vi "HCCDiceTester.vi"(11 "COM Port MicroZed":refnum<visa-resource-name>="COM4") -> ()   [LabVIEW 2014]
uses:
  c_StateMachine_States.ctl
  <vilib>/vision/Vision Builder AI/API.llb/IVB Interface - VBAI Version.ctl
  c_VBAI_SelcectInspection.ctl
  c_PlatePosEnum.ctl
  c_InstructionEnum.ctl
  c_Calib_States.ctl
  c_ShowCorner_States.ctl
  c_FindReference_States.ctl
  c_ReportMessages.ctl
  g_Stop.vi
  g_ReportControl.vi
  g_GPCounters.vi
  g_CipHolderConstants.vi
  g_CommandParam.vi
  g_VBAIMeasurements.vi
  g_MicroZed_Interface.vi
  g_ChipData.vi
  g_ImageCalibration.vi
  g_HCCConstants.vi
panel:
  in  "RedoAlignment":bool
  out "Chip Y":dbl
  out "Chip X":dbl
  in  "BrightnessAdjustment":bool
  in  "Move Plate":bool
  out "Alignment Successful":bool
  in  "CancelAlignment":bool
  in  "ConfirmAlignment":bool
  in  "ProbecardOK":bool
  out "ChipsComplete":bool
  out "LoopBreak":bool
  in  "ImageBusy":bool
  in  "stop":bool
  out "Image":T1(plugin-control)
  out "Actual State":T2
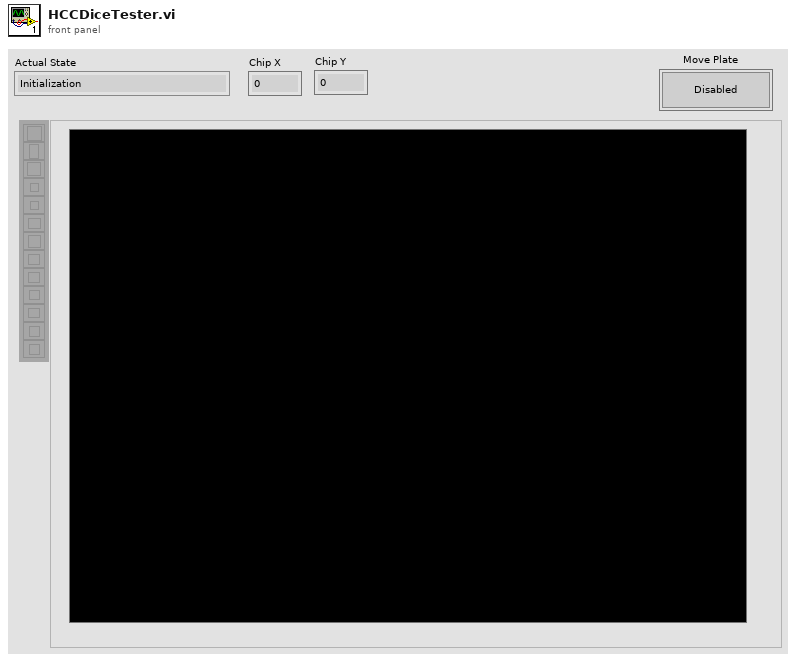
[diagram p1: front panel]
types:
  T1 = typedef "IMAQ Image.ctl" = refnum<image>
  T2 = typedef "c_StateMachine_States.ctl" = enum16{"Initialization", "Load", "Calibration", "Next Slot", "Chip Alignment", "Test", "Report", "End"}
  T3 = enum8{"Enabled", "Disabled", "Disabled and Grayed Out"}
  T4 = typedef "IVB Interface - VBAI Version.ctl" = u16
  T5 = enum32{"invalid app kind", "Development System", "Run Time System", "Student Edition", "Embedded LabVIEW", "Evaluation", "Custom"}
  T6 = typedef "VBAIInterface.ctl" = refnum<k21>
  T7 = typedef "c_InstructionEnum.ctl" = enum16{"Move Absolute", "Increment", "Move Home", "Motion Kill", "Move Plate", "Set Stepsize", "Query Position"}
  T8 = typedef "c_PlatePosEnum.ctl" = enum16{"Contact", "Seperate"}
  T9 = typedef "c_VBAI_SelcectInspection.ctl" = enum16{"Image Acquisition", "Find Reference", "Chip Alignment", "Adjustment", "Porbecard Positioning"}
  T10 = typedef "c_Calib_States.ctl" = enum16{"Find Top", "Show Corners", "Find Reference"}
  T11 = typedef "c_ShowCorner_States.ctl" = enum16{"Intruction", "Set Increment", "First Move Right", "Move Right", "Move Left", "Confirm"}
  T12 = typedef "c_FindReference_States.ctl" = enum16{"Move to Side", "Settings", "Find Chipslot", "Make Step", "Set Reference"}
  T13 = typedef "c_ReportMessages.ctl" = string
  T14 = cluster{"PASS/FAIL Flag":bool, "Numeric Measurement":dbl, "String Measurement":string, "Report Text":string}
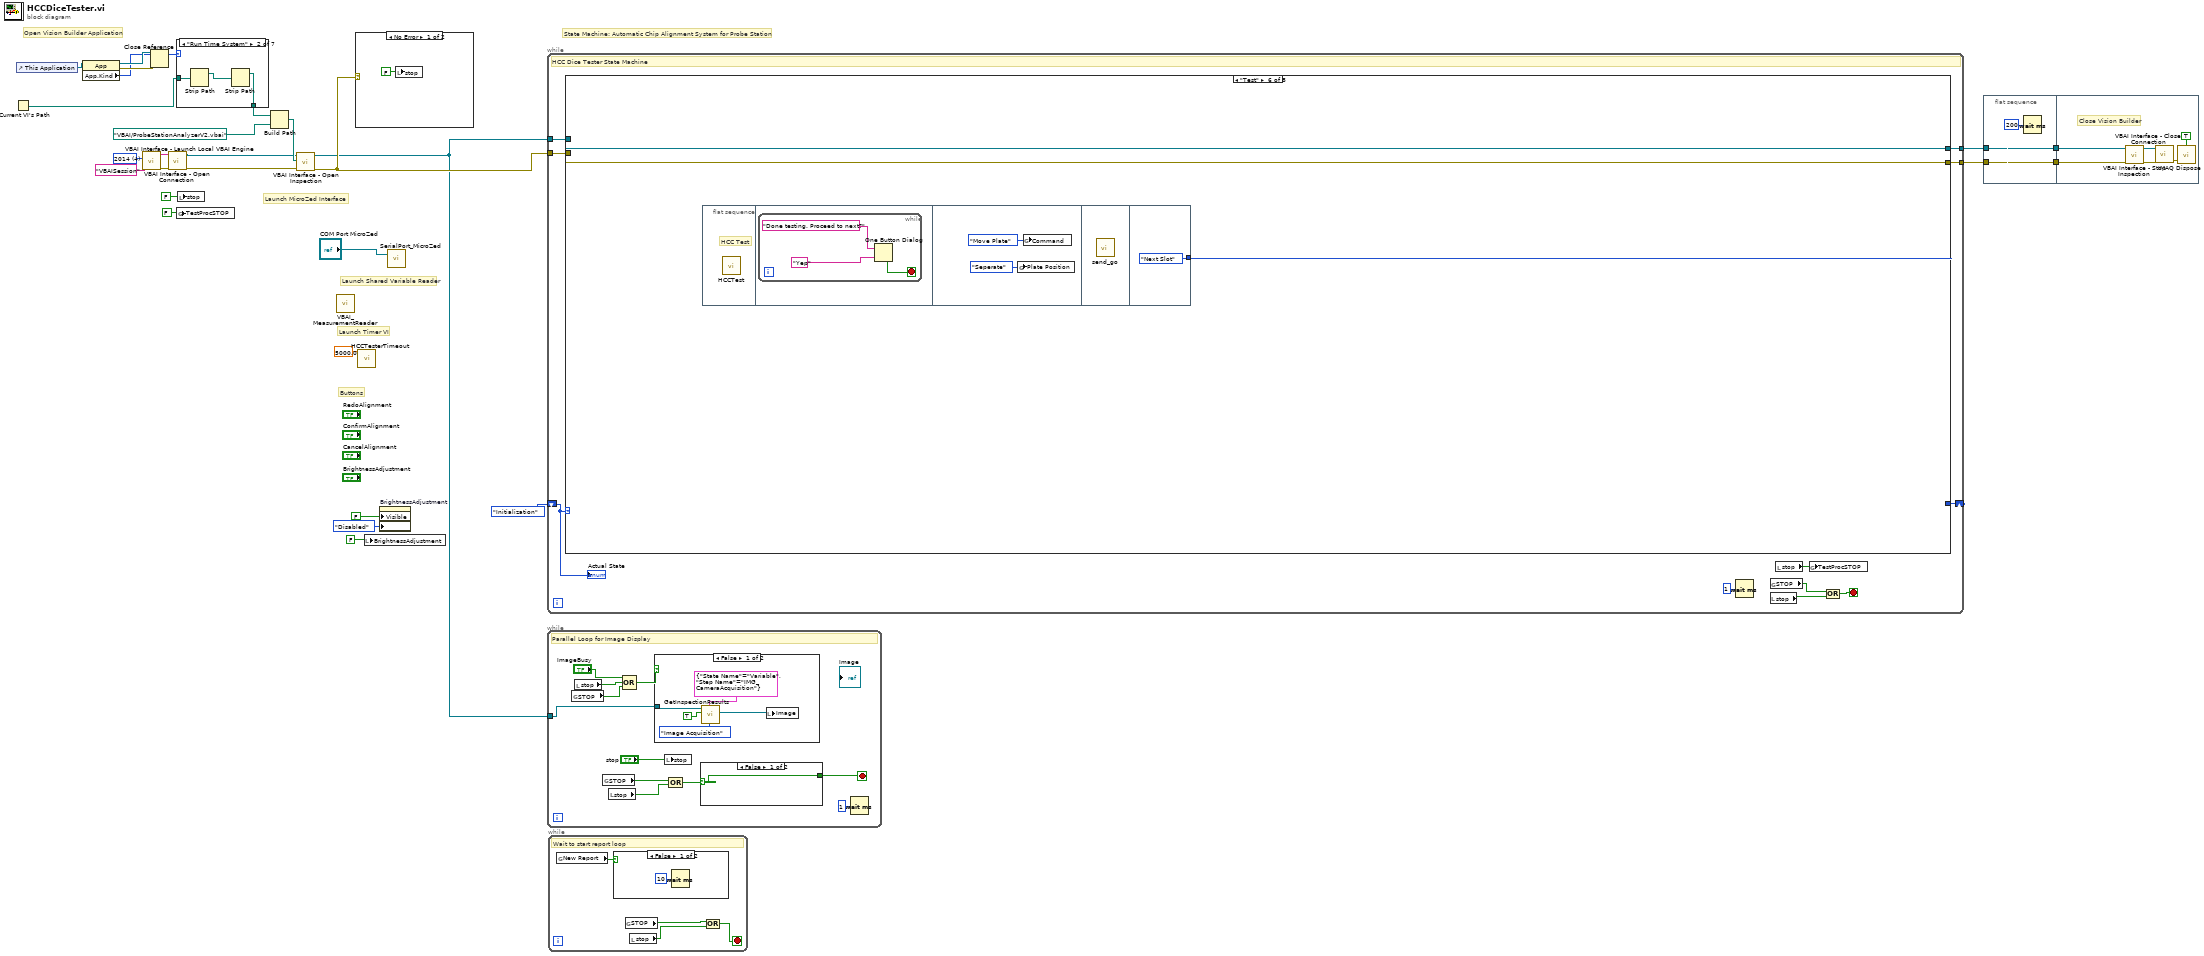
[diagram p0: block diagram]
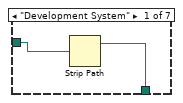
[diagram p2: hidden frame]
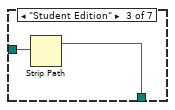
[diagram p3: hidden frame]
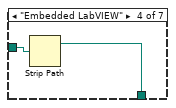
[diagram p4: hidden frame]
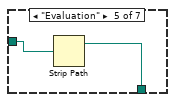
[diagram p5: hidden frame]
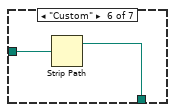
[diagram p6: hidden frame]
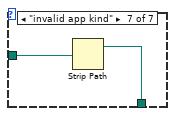
[diagram p7: hidden frame]
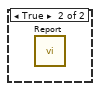
[diagram p8: hidden frame]
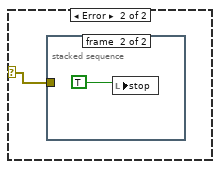
[diagram p9: hidden frame]
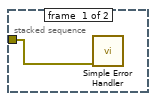
[diagram p10: hidden frame]
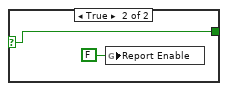
[diagram p11: hidden frame]
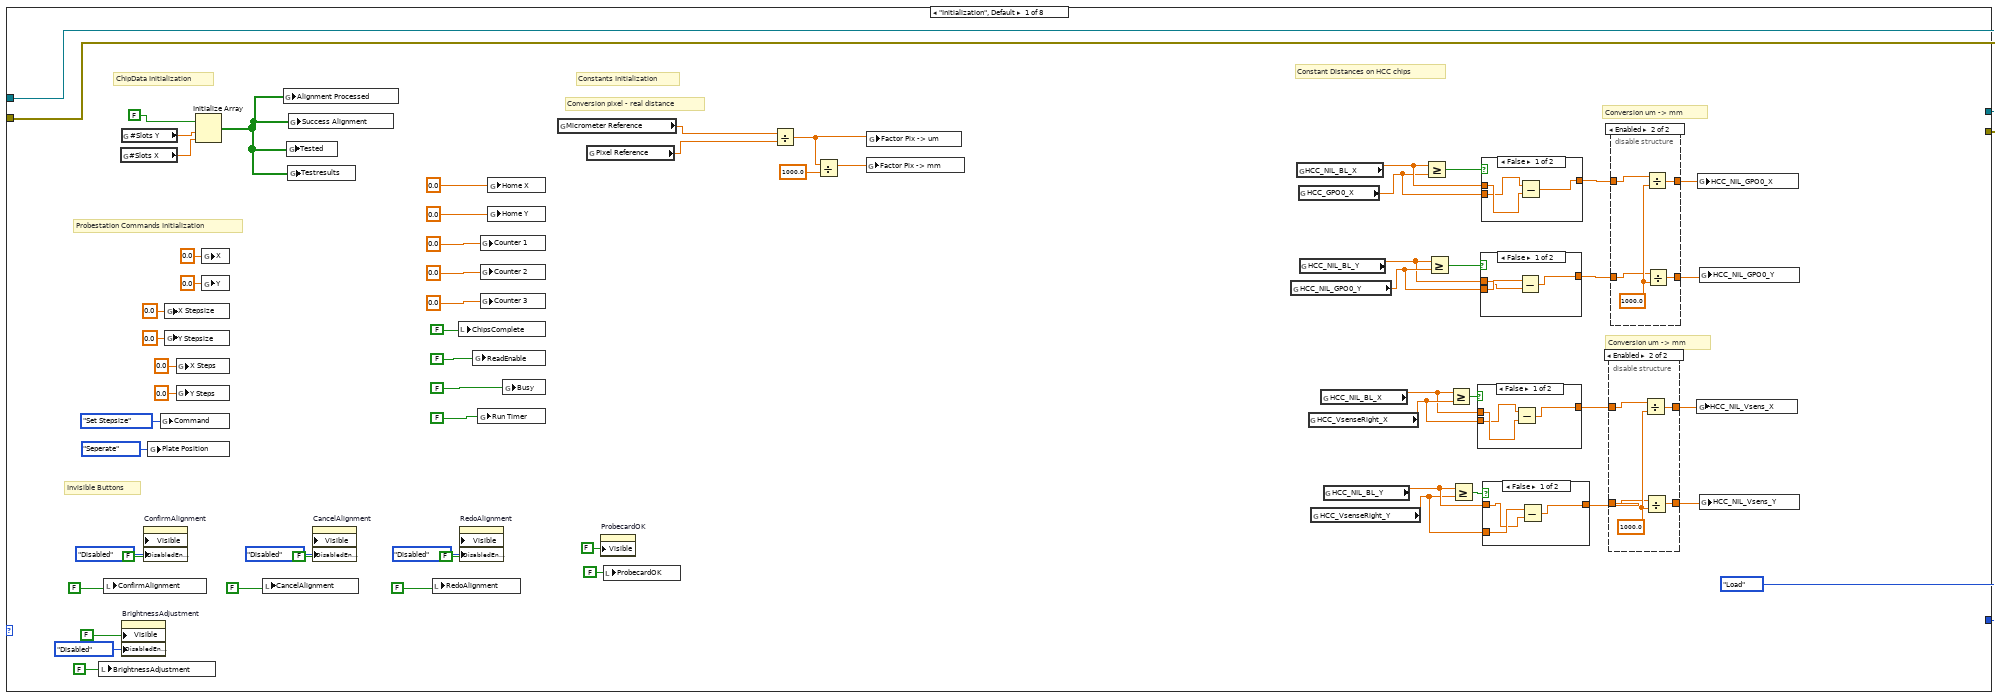
[diagram p13: hidden frame]
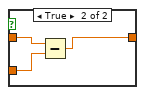
[diagram p15: hidden frame]
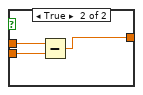
[diagram p16: hidden frame]
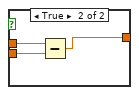
[diagram p18: hidden frame]
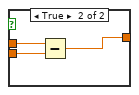
[diagram p19: hidden frame]
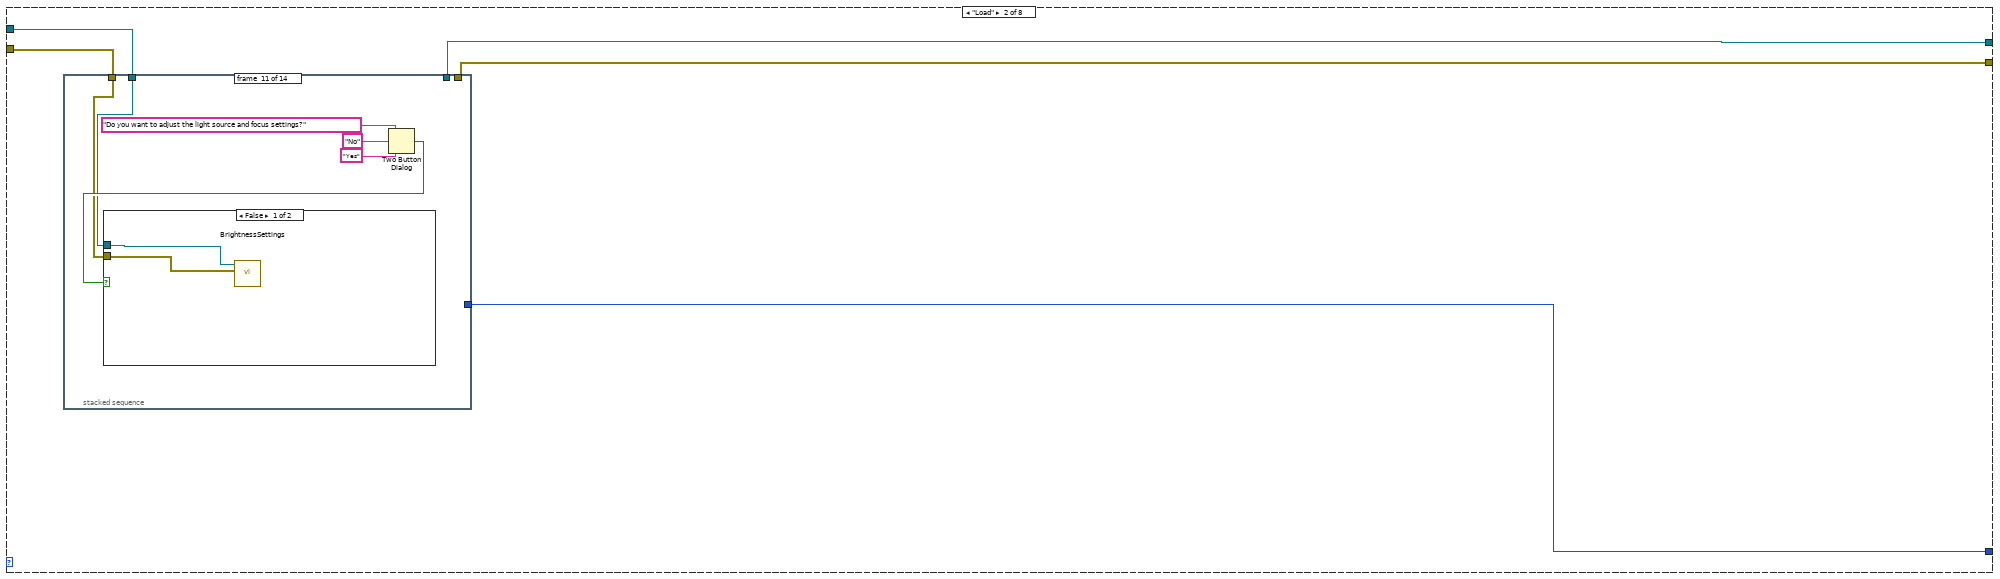
[diagram p20: hidden frame]
diagram:
  w27 = T4 4 items=["2010", "2011", "2012", "2013", "2014"] ("Engine Version")
  # "Buttons"
  # "Launch Timer VI"
  # "Launch Shared Variable Reader"
  # "Launch MicroZed Interface"
  # "Open Vision Builder Application"
  # "State Machine: Automatic Chip Alignment System for Probe Station"
  n1 = Current VI's Path() -> (path=w5:path)
  n2 = control-ref of="This Application"() -> (w7:refnum<vi>)
  n3 = property class="App"(reference=w7) -> (reference out=w9:refnum<vi>, error out=w8:errorcluster, "App.Kind"=w6:T5)  [unwired: 1 in]
  n4 = call <vilib>:"VBAI Interface - Launch Local VBAI Engine.vi"("Engine Version"=w27, "Local VBAI Engine Name"="VBAISession") -> ("error out"=w26:errorcluster, "Session Name Out"=w25:string)  [unwired: 8 in]
  n5 = Close Reference(reference=w9, error in (no error)=w8) -> ()  [unwired: 1 out]
  n6 = call <vilib>:"VBAI Interface - Open Connection.vi"("error in"=w26, "Session In"=w25) -> ("error out"=w20:errorcluster, "Session Out"=w21:T6)  [unwired: 8 in]
  n7 = case shown="\"Run Time System\"" w6 {
    tunnel: w5 -> [w30 w33 w35 w37 w39 w41 w42]
    tunnel: [w29 w31 w34 w36 w38 w40 w43] -> w4
    frame "Development System" {
      n8 = Strip Path(path=w30) -> (stripped path=w29:path)  [unwired: 1 out]
    }
    frame "Run Time System" {
      n9 = Strip Path(path=w33) -> (stripped path=w32:path)  [unwired: 1 out]
      n10 = Strip Path(path=w32) -> (stripped path=w31:path)  [unwired: 1 out]
    }
    frame "Student Edition" {
      n11 = Strip Path(path=w35) -> (stripped path=w34:path)  [unwired: 1 out]
    }
    frame "Embedded LabVIEW" {
      n12 = Strip Path(path=w37) -> (stripped path=w36:path)  [unwired: 1 out]
    }
    frame "Evaluation" {
      n13 = Strip Path(path=w39) -> (stripped path=w38:path)  [unwired: 1 out]
    }
    frame "Custom" {
      n14 = Strip Path(path=w41) -> (stripped path=w40:path)  [unwired: 1 out]
    }
    frame "invalid app kind" {
      n15 = Strip Path(path=w42) -> (stripped path=w43:path)  [unwired: 1 out]
    }
  }
  n16 = global write "g_Stop.vi" "TestProcSTOP"(FALSE ("TestProcSTOP")) -> ()
  n17 = local write "stop"(FALSE ("stop")) -> ()
  n18 = Build Path(base path=w4, name or relative path=path "VBAI/ProbeStationAnalyzerV2.vbai") -> (appended path=w22:path)
  n19 = call <vilib>:"VBAI Interface - Open Inspection.vi"("error in"=w20, "Path"=w22, "Session In"=w21) -> ("error out"=w17:errorcluster, "Session Out"=w16:T6)  [unwired: 7 in]
  n20 = call "VBAI_MeasurementReader.vi"() -> ()  [unwired: 12 in]
  n21 = case shown="No Error" w17 {
    selector: w17 -> [_ w45]
    frame No Error {
      n22 = local write "stop"(FALSE) -> ()
    }
    frame Error {
      n23 = stacked-sequence {
        tunnel: w45 -> [w46 _]
        frame #0 {
          n24 = call <vilib>:"Simple Error Handler.vi"("error in (no error)"=w46) -> ()  [unwired: 4 in, 5 out]
        }
        frame #1 {
          n25 = local write "stop"(TRUE) -> ()
        }
      }
    }
  }
  n26 = call "HCCTesterTimeout.vi"("Timeout"=5000.0) -> ()  [unwired: 11 in]
  n27 = local write "BrightnessAdjustment"(FALSE ("CancelAlignment")) -> ()
  n28 = property on="BrightnessAdjustment" class="Bool (strict)"("Visible"=FALSE, "DisabledEnum"=T3."Disabled" ("Disabled")) -> ()  [unwired: 2 in, 2 out]
  n29 = call "SerialPort_MicroZed.vi"("COM Port"="COM Port MicroZed") -> ()  [unwired: 2 in, 1 out]
  n30 = while {
    shift-right: [w58] -> _
    shift-left: c_StateMachine_States."Initialization" -> [w48]
    tunnel: w16 -> [w54]
    tunnel: w17 -> [w52]
    tunnel: [w55] -> w19
    tunnel: [w53] -> w18
    stop <- w56 stop-if-true
    # "HCC Dice Tester State Machine"
    n31 = case shown="\"Test\"" w48 {
      tunnel: [c_StateMachine_States."Load" w164 c_StateMachine_States."Next Slot" w433 w499 w639 c_StateMachine_States."End" c_StateMachine_States."End"] -> w58
      tunnel: [w67 w161 w207 w435 w503 w641 w651 w664] -> w55
      tunnel: w54 -> [w67 w162 w209 w435 w505 w641 w651 w664]
      tunnel: [w66 w160 w206 w434 w502 w640 w650 w663] -> w53
      tunnel: w52 -> [w66 w163 w208 w434 w504 w640 w650 w663]
      frame "Initialization", Default {
        # "Constant Distances on HCC chips"
        # "Invisible Buttons"
        # "Conversion pixel - real distance"
        # "Probestation Commands Initialization"
        # "Conversion um -> mm"
        # "Conversion um -> mm"
        # "Constants Initialization"
        # "ChipData Initialization"
        n32 = local write "BrightnessAdjustment"(FALSE ("CancelAlignment")) -> ()
        n33 = local write "ConfirmAlignment"(FALSE ("ConfirmAlignment")) -> ()
        n34 = global read "g_CipHolderConstants.vi" "#Slots X"() -> (w120:dbl)
        n35 = global read "g_CipHolderConstants.vi" "#Slots Y"() -> (w121:dbl)
        n36 = property on="BrightnessAdjustment" class="Bool (strict)"("Visible"=FALSE, "DisabledEnum"=T3."Disabled" ("Disabled")) -> ()  [unwired: 2 in, 2 out]
        n37 = property on="ConfirmAlignment" class="Bool (strict)"("Visible"=FALSE, "DisabledEnum"=T3."Disabled" ("Disabled")) -> ()  [unwired: 2 in, 2 out]
        n38 = global write "g_CommandParam.vi" "Plate Position"(c_PlatePosEnum."Seperate" ("Plate Position")) -> ()
        n39 = global write "g_CommandParam.vi" "Command"(c_InstructionEnum."Set Stepsize" ("Command")) -> ()
        n40 = global write "g_CommandParam.vi" "X Stepsize"(0.0 ("X Stepsize")) -> ()
        n41 = global write "g_CommandParam.vi" "Y Stepsize"(0.0 ("Y Stepsize")) -> ()
        n42 = global write "g_CommandParam.vi" "X Steps"(0.0 ("X Steps")) -> ()
        n43 = global write "g_CommandParam.vi" "Y Steps"(0.0 ("Y Steps")) -> ()
        n44 = Initialize Array(FALSE, w121, w120) -> (w79:bool[][])
        n45 = global write "g_CommandParam.vi" "X"(0.0 ("X")) -> ()
        n46 = global write "g_CommandParam.vi" "Y"(0.0 ("Y")) -> ()
        n47 = local write "CancelAlignment"(FALSE ("CancelAlignment")) -> ()
        n48 = global write "g_ChipData.vi" "Alignment Processed"(w79) -> ()
        n49 = global write "g_ChipData.vi" "Tested"(w79) -> ()
        n50 = global write "g_ChipData.vi" "Testresults"(w79) -> ()
        n51 = global write "g_ChipData.vi" "Success Alignment"(w79) -> ()
        n52 = property on="CancelAlignment" class="Bool (strict)"("Visible"=FALSE, "DisabledEnum"=T3."Disabled" ("Disabled")) -> ()  [unwired: 2 in, 2 out]
        n53 = local write "RedoAlignment"(FALSE ("CancelAlignment")) -> ()
        n54 = local write "ChipsComplete"(FALSE ("ChipsComplete")) -> ()
        n55 = property on="RedoAlignment" class="Bool (strict)"("Visible"=FALSE ("RedoAlignment"), "DisabledEnum"=T3."Disabled" ("RedoAlignment")) -> ()  [unwired: 2 in, 2 out]
        n56 = global write "g_VBAIMeasurements.vi" "ReadEnable"(FALSE ("SharedVariableReadEnable")) -> ()
        n57 = global write "g_MicroZed_Interface.vi" "Run Timer"(FALSE ("Start")) -> ()
        n58 = global write "g_GPCounters.vi" "Counter 1"(0.0 ("Counter 1")) -> ()
        n59 = global write "g_GPCounters.vi" "Counter 2"(0.0 ("Counter 1")) -> ()
        n60 = global write "g_GPCounters.vi" "Counter 3"(0.0 ("Counter 1")) -> ()
        n61 = global write "g_CipHolderConstants.vi" "Home X"(0.0 ("Home X")) -> ()
        n62 = global write "g_CipHolderConstants.vi" "Home Y"(0.0 ("Home X")) -> ()
        n63 = global write "g_MicroZed_Interface.vi" "Busy"(FALSE ("Busy")) -> ()
        n64 = global read "g_ImageCalibration.vi" "Micrometer Reference"() -> (w111:dbl)
        n65 = global read "g_ImageCalibration.vi" "Pixel Reference"() -> (w112:dbl)
        n66 = property on="ProbecardOK" class="Bool (strict)"("Visible"=FALSE) -> ()  [unwired: 2 in, 2 out]
        n67 = local write "ProbecardOK"(FALSE ("ProbecardOK")) -> ()
        n68 = Divide(x=w111, y=w112) -> (x/y=w110:dbl)
        n69 = Divide(x=w110, y=1000.0) -> (x/y=w108:dbl)
        n70 = global write "g_ImageCalibration.vi" "Factor Pix -> mm"(w108) -> ()
        n71 = global write "g_ImageCalibration.vi" "Factor Pix -> um"(w110) -> ()
        n72 = global read "g_HCCConstants.vi" "HCC_NIL_GPO0_Y"() -> (w104:dbl)
        n73 = global read "g_HCCConstants.vi" "HCC_NIL_BL_X"() -> (w106:dbl)
        n74 = global read "g_HCCConstants.vi" "HCC_GPO0_X"() -> (w105:dbl)
        n75 = global read "g_HCCConstants.vi" "HCC_NIL_BL_Y"() -> (w103:dbl)
        n76 = global read "g_HCCConstants.vi" "HCC_VsenseRight_X"() -> (w90:dbl)
        n77 = global read "g_HCCConstants.vi" "HCC_VsenseRight_Y"() -> (w91:dbl)
        n78 = global read "g_HCCConstants.vi" "HCC_NIL_BL_X"() -> (w89:dbl)
        n79 = global read "g_HCCConstants.vi" "HCC_NIL_BL_Y"() -> (w92:dbl)
        n80 = Greater Or Equal?(x=w106, y=w105) -> (x >= y?=w107:bool)
        n81 = Greater Or Equal?(x=w103, y=w104) -> (x >= y?=w102:bool)
        n82 = Greater Or Equal?(x=w89, y=w90) -> (x >= y?=w88:bool)
        n83 = Greater Or Equal?(x=w92, y=w91) -> (x >= y?=w93:bool)
        n84 = case shown="False" w88 {
          tunnel: w89 -> [w136 w140]
          tunnel: w90 -> [w135 w139]
          tunnel: [w137 w138] -> w94
          frame False {
            n85 = Subtract(x=w135, y=w136) -> (x-y=w137:dbl)
          }
          frame True {
            n86 = Subtract(x=w140, y=w139) -> (x-y=w138:dbl)
          }
        }
        n87 = case shown="False" w102 {
          tunnel: w103 -> [w148 w153]
          tunnel: w104 -> [w149 w152]
          tunnel: [w150 w151] -> w99
          frame False {
            n88 = Subtract(x=w149, y=w148) -> (x-y=w150:dbl)
          }
          frame True {
            n89 = Subtract(x=w153, y=w152) -> (x-y=w151:dbl)
          }
        }
        n90 = case shown="False" w107 {
          tunnel: w106 -> [w155 w159]
          tunnel: w105 -> [w154 w158]
          tunnel: [w156 w157] -> w101
          frame False {
            n91 = Subtract(x=w154, y=w155) -> (x-y=w156:dbl)
          }
          frame True {
            n92 = Subtract(x=w159, y=w158) -> (x-y=w157:dbl)
          }
        }
        n93 = case shown="False" w93 {
          tunnel: w92 -> [w129 w133]
          tunnel: w91 -> [w130 w132]
          tunnel: [w131 w134] -> w96
          frame False {
            n94 = Subtract(x=w130, y=w129) -> (x-y=w131:dbl)
          }
          frame True {
            n95 = Subtract(x=w133, y=w132) -> (x-y=w134:dbl)
          }
        }
        n96 = disable-structure shown="Enabled" {
          disable-tunnel: w94 -> [w123 w125]
          disable-tunnel: [w123 w128] -> w95
          disable-tunnel: w96 -> [w122 w124]
          disable-tunnel: [w122 w127] -> w97
          frame Disabled {
          }
          frame Enabled {
            w126 = 1000.0 ("y")
            n97 = Divide(x=w125, y=w126) -> (x/y=w128:dbl)
            n98 = Divide(x=w124, y=w126) -> (x/y=w127:dbl)
          }
        }
        n99 = disable-structure shown="Enabled" {
          disable-tunnel: w101 -> [w142 w144]
          disable-tunnel: [w142 w147] -> w100
          disable-tunnel: w99 -> [w141 w143]
          disable-tunnel: [w141 w146] -> w98
          frame Disabled {
          }
          frame Enabled {
            w145 = 1000.0 ("y")
            n100 = Divide(x=w144, y=w145) -> (x/y=w147:dbl)
            n101 = Divide(x=w143, y=w145) -> (x/y=w146:dbl)
          }
        }
        n102 = global write "g_HCCConstants.vi" "HCC_NIL_Vsens_X"(w95) -> ()
        n103 = global write "g_HCCConstants.vi" "HCC_NIL_GPO0_X"(w100) -> ()
        n104 = global write "g_HCCConstants.vi" "HCC_NIL_GPO0_Y"(w98) -> ()
        n105 = global write "g_HCCConstants.vi" "HCC_NIL_Vsens_Y"(w97) -> ()
      }
      frame "Load" {
        n106 = stacked-sequence {
          tunnel: w162 -> [_ _ _ _ _ _ _ _ w179 _ w194 _ _ _]
          tunnel: w163 -> [_ _ _ _ _ _ _ _ w178 _ w193 _ _ _]
          tunnel: [_ _ _ _ _ _ _ _ _ _ _ _ _ c_StateMachine_States."Calibration"] -> w164
          tunnel: [_ _ _ _ _ _ _ _ w177 _ _ _ _ _] -> w161
          tunnel: [_ _ _ _ _ _ _ _ w176 _ _ _ _ _] -> w160
          frame #0 {
            n107 = global write "g_CommandParam.vi" "Command"(c_InstructionEnum."Move Absolute" ("Command")) -> ()
            n108 = call "send_go.vi"() -> ()  [unwired: 12 in]
            n109 = global write "g_CommandParam.vi" "X"(0.0 ("X")) -> ()
            n110 = global write "g_CommandParam.vi" "Y"(70.0 ("Y")) -> ()
          }
          frame #1 {
            n111 = One Button Dialog(message="Place the Chips on the Chipholder and click OK") -> ()  [unwired: 1 in, 1 out]
          }
          frame #2 {
            # "Select the chipslots that are\noccupied by a chip"
            n112 = call "ChipSlotSelect.vi"() -> ()  [unwired: 12 in]
          }
          frame #3 {
            # "Start a new report dialog"
            n113 = global write "g_ReportControl.vi" "New Report"(TRUE ("New Report")) -> ()
          }
          frame #4 {
            n114 = Wait (ms)(milliseconds to wait=u32 1) -> ()  [unwired: 1 out]
          }
          frame #5 {
            # "Wait until new report dialog ended"
            n115 = while {
              stop <- w172 stop-if-true
              n116 = global read "g_ReportControl.vi" "New Report"() -> (w173:bool)
              n117 = Not(x=w173) -> (.not. x?=w172:bool)
              n118 = Wait (ms)(milliseconds to wait=u32 100) -> ()  [unwired: 1 out]
            }
          }
          frame #6 {
            # "Set the Configurationregisters\nfor the HCC chips"
            n119 = call "HCCConfig.vi"() -> ()  [unwired: 12 in]
          }
          frame #7 {
            # "Propare for Image Processing\n- Set Image Busy\n- Make Button visible for\nProbecard Alignment Confirm"
            n120 = local write "ImageBusy"(TRUE ("ImageBusy")) -> ()
            n121 = property on="ProbecardOK" class="Bool (strict)"("Visible"=TRUE) -> ()  [unwired: 2 in, 2 out]
          }
          frame #8 {
            # "Show Probecard Highlight until Confirm"
            n122 = while {
              tunnel: [w189] -> w177
              tunnel: w178 -> [w182]
              tunnel: [w188] -> w176
              tunnel: w179 -> [w183]
              stop <- w185 stop-if-true
              n123 = global read "g_Stop.vi" "TestProcSTOP"() -> (w187:bool)
              n124 = global read "g_Stop.vi" "STOP"() -> (w186:bool)
              n125 = call "GetInspectionResults.vi"("Select Inspection"=c_VBAI_SelcectInspection."Porbecard Positioning" ("Enum"), "Image Step Name (default last image used by inspection)"=cluster{"State Name":string, "Step Name":string} {"State Name"="Variable", "Step Name"="IMG_ProbeCardPosition"}, "error in (no error)"=w182, "Image Enable"=TRUE, "Refnum in"=w183) -> ("error out"=w188:errorcluster, "Image Dst Out"=w181:T1, "Refnum out"=w189:T6)  [unwired: 2 in, 2 out]
              n126 = Compound Arithmetic op=OR("ProbecardOK", w186, w187) -> (w185:bool)
              n127 = local write "Image"(w181) -> ()
            }
          }
          frame #9 {
            # "Hide Button again and\nfree image for normal Display"
            n128 = property on="ProbecardOK" class="Bool (strict)"("Visible"=FALSE) -> ()  [unwired: 2 in, 2 out]
          }
          frame #10 {
            n129 = Two Button Dialog(message="Do you want to adjust the light source and focus settings?", 1:"Yes" ("F button name (\"Cancel\")"), 2:"No" ("T button name (\"OK\")")) -> (T button?=w195:bool)
            n130 = case shown="False" w195 {
              tunnel: w194 -> [w200 _]
              tunnel: w193 -> [w199 _]
              frame False {
                n131 = call "BrightnessSettings.vi"("error in (no error)"=w199, "Refnum in"=w200) -> ()  [unwired: 8 in, 2 out]
              }
              frame True {
              }
            }
          }
          frame #11 {
            n132 = Wait (ms)(milliseconds to wait=u32 100) -> ()  [unwired: 1 out]
          }
          frame #12 {
            n133 = disable-structure shown="Disabled" {
              frame Disabled {
                n134 = local write "ImageBusy"(FALSE ("ImageBusy")) -> ()
              }
              frame Enabled {
              }
            }
          }
          frame #13 {
          }
        }
      }
      frame "Calibration" {
        n135 = while {
          shift-right: [w210] -> _
          shift-left: c_Calib_States."Find Top" -> [w213]
          tunnel: w209 -> [w218]
          tunnel: w208 -> [w217]
          tunnel: [w216] -> w207
          tunnel: [w215] -> w206
          stop <- w214 stop-if-true
          # "Calibration State Machine"
          n136 = case shown="\"Find Reference\"" w213 {
            tunnel: [FALSE FALSE TRUE] -> w211
            tunnel: [w223 c_Calib_States."Find Reference" c_Calib_States."Find Reference"] -> w210
            tunnel: w218 -> [w225 w288 w341]
            tunnel: w217 -> [w224 w290 w340]
            tunnel: [w222 w288 w338] -> w216
            tunnel: [w221 w290 w337] -> w215
            frame "Find Top", Default {
              n137 = stacked-sequence {
                tunnel: w225 -> [_ _ _ _ _ _ w248 _]
                tunnel: w224 -> [_ _ _ _ _ _ w247 _]
                tunnel: [_ _ _ _ _ _ w246 _] -> w222
                tunnel: [_ _ _ _ _ _ w245 _] -> w221
                tunnel: [_ _ _ _ _ _ _ c_Calib_States."Show Corners"] -> w223
                frame #0 {
                  n138 = Wait (ms)(milliseconds to wait=u32 1) -> ()  [unwired: 1 out]
                }
                frame #1 {
                  # "Move back from the Load Position towards the\nregion of the chipholder"
                  n139 = global read "g_CipHolderConstants.vi" "Length Chipslot"() -> (w232:dbl)
                  n140 = global read "g_CipHolderConstants.vi" "#Slots Y"() -> (w231:dbl)
                  n141 = global write "g_CommandParam.vi" "Command"(c_InstructionEnum."Move Absolute" ("Command")) -> ()
                  n142 = global write "g_CommandParam.vi" "X"(0.0 ("X")) -> ()
                  n143 = Multiply(x=w231, y=w232) -> (x*y=w233:dbl)
                  n144 = Divide(x=w233, y=2.0) -> (x/y=w230:dbl)
                  n145 = Multiply(x=w230, y=1.0) -> (x*y=w229:dbl)
                  n146 = global write "g_CommandParam.vi" "Y"(w229) -> ()
                }
                frame #2 {
                  # "Send Command"
                  n147 = call "send_go.vi"() -> ()  [unwired: 12 in]
                }
                frame #3 {
                  # "Wait during movement"
                  n148 = Wait (ms)(milliseconds to wait=u32 1500) -> ()  [unwired: 1 out]
                }
                frame #4 {
                  # "Wait until Probestation is ready"
                  n149 = call "PS_Ready.vi"("WaitForReady"=TRUE) -> ()  [unwired: 10 in, 1 out]
                }
                frame #5 {
                  n150 = flat-sequence {
                    frame #0 {
                      # "Prepare to find Top Edge\n- Set Stepsize\n- Set Image Busz for Image Processing\n- Set maximal Stepcounter to 0"
                      n151 = global write "g_GPCounters.vi" "Counter 2"(0.0 ("Counter 2")) -> ()
                      n152 = global write "g_CommandParam.vi" "Y Stepsize"(0.1 ("Y Stepsize")) -> ()
                      n153 = local write "ImageBusy"(TRUE ("ImageBusy")) -> ()
                      n154 = global write "g_CommandParam.vi" "X Stepsize"(0.1 ("X Stepsize")) -> ()
                      n155 = global write "g_CommandParam.vi" "Command"(c_InstructionEnum."Set Stepsize" ("Command")) -> ()
                    }
                    frame #1 {
                    }
                    frame #2 {
                      n156 = call "send_go.vi"() -> ()  [unwired: 12 in]
                    }
                    frame #3 {
                      n157 = call "send_go.vi"() -> ()  [unwired: 12 in]
                    }
                    frame #4 {
                      n158 = Wait (ms)(milliseconds to wait=u32 1) -> ()  [unwired: 1 out]
                    }
                  }
                }
                frame #6 {
                  n159 = while {
                    tunnel: w248 -> [w264]
                    tunnel: w247 -> [w263]
                    tunnel: [w262] -> w246
                    tunnel: [w261] -> w245
                    stop <- w269 stop-if-true
                    # "Stops the Loop when more than 50 moves executed\nchange steps from 40 to 50 8/19/15 -nl"
                    # "Edge Detection\nLooking for Top Edge of \nthe Chipholder"
                    # "This Loop moves the chuck until the top edge of the chipholder is detected"
                    n160 = call "GetInspectionResults.vi"("Select Inspection"=c_VBAI_SelcectInspection."Find Reference", "Image Step Name (default last image used by inspection)"=cluster{"State Name":string, "Step Name":string} {"State Name"="Variable", "Step Name"="IMG_EdgeFinder"}, "error in (no error)"=w263, "StepName"="FindTop", "Image Enable"=TRUE, "Refnum in"=w264) -> ("error out"=w261:errorcluster, "Results"=w267:T14, "Image Dst Out"=w260:T1, "Refnum out"=w262:T6)  [unwired: 1 in, 1 out]
                    n161 = local write "Image"(w260) -> ()
                    n162 = Unbundle By Name(w267) -> ("PASS/FAIL Flag"=w250:bool)
                    n163 = case shown="False" w250 {
                      frame False {
                        # "If no Edge detected -> Move a step"
                        n164 = stacked-sequence {
                          frame #0 {
                            n165 = global read "g_GPCounters.vi" "Counter 2"() -> (w274:dbl)
                            n166 = global write "g_GPCounters.vi" "Counter 1"(0.0 ("Counter 1")) -> ()
                            n167 = Increment(x=w274) -> (x+1=w275:dbl)
                            n168 = global write "g_GPCounters.vi" "Counter 2"(w275) -> ()
                          }
                          frame #1 {
                            n169 = global write "g_CommandParam.vi" "Y Stepsize"(0.1 ("Y Stepsize")) -> ()
                            n170 = global write "g_CommandParam.vi" "X Stepsize"(0.1 ("X Stepsize")) -> ()
                            n171 = global write "g_CommandParam.vi" "Command"(c_InstructionEnum."Set Stepsize" ("Command")) -> ()
                          }
                          frame #2 {
                            n172 = call "send_go.vi"() -> ()  [unwired: 12 in]
                          }
                          frame #3 {
                            n173 = global write "g_CommandParam.vi" "Y Steps"(-1.0 ("Y Stepsize")) -> ()
                            n174 = global write "g_CommandParam.vi" "X Steps"(0.0 ("X Stepsize")) -> ()
                            n175 = global write "g_CommandParam.vi" "Command"(c_InstructionEnum."Increment" ("Command")) -> ()
                          }
                          frame #4 {
                            n176 = call "send_go.vi"() -> ()  [unwired: 12 in]
                          }
                          frame #5 {
                            n177 = Wait (ms)(milliseconds to wait=200) -> ()  [unwired: 1 out]
                          }
                        }
                      }
                      frame True {
                        # "If Edge is detected, repeat to be sure that\nEdge is still detected and it is not \njust a random detection"
                        n178 = global read "g_GPCounters.vi" "Counter 1"() -> (w285:dbl)
                        n179 = Increment(x=w285) -> (x+1=w284:dbl)
                        n180 = global write "g_GPCounters.vi" "Counter 1"(w284) -> ()
                      }
                    }
                    n181 = global read "g_GPCounters.vi" "Counter 2"() -> (w253:dbl)
                    n182 = global read "g_GPCounters.vi" "Counter 1"() -> (w257:dbl)
                    n183 = Greater?(x=w257, y=3.0) -> (0:w255:bool)
                    n184 = Greater?(x=w253, y=100.0) -> (0:w251:bool)
                    n185 = case shown="True" w251 {
                      tunnel: [FALSE ("stop") w271] -> w249
                      frame False {
                      }
                      frame True {
                        n186 = stacked-sequence {
                          tunnel: [_ w273] -> w271
                          frame #0 {
                            n187 = One Button Dialog(message="Chipholder not found! Click OK and restart the Testprocedure") -> ()  [unwired: 1 in, 1 out]
                          }
                          frame #1 {
                            w273 = TRUE ("stop")
                            n188 = local write "stop"(w273) -> ()
                          }
                        }
                      }
                    }
                    n189 = global read "g_Stop.vi" "STOP"() -> (w268:bool)
                    n190 = local read "stop"() -> (w259:bool)
                    n191 = Compound Arithmetic op=OR(w249, w268, w255, w259) -> (w269:bool)
                  }
                }
                frame #7 {
                  # "Free Image for normal Display"
                  n192 = local write "ImageBusy"(FALSE ("ImageBusy")) -> ()
                }
              }
            }
            frame "Show Corners" {
              n193 = while {
                shift-right: [w297] -> _
                shift-left: c_ShowCorner_States."Intruction" -> [w298]
                stop <- w294 stop-if-true
                # "Show Corners State Machine"
                n194 = case shown="\"First Move Right\"" w298 {
                  tunnel: [c_ShowCorner_States."Set Increment" w302 c_ShowCorner_States."Move Left" c_ShowCorner_States."Move Left" c_ShowCorner_States."Confirm" w330] -> w297
                  tunnel: [FALSE ("T button?") _ _ _ _ w331] -> w293
                  frame "Intruction", Default {
                    # "Instruction for the user"
                    n195 = One Button Dialog(message="The chuck will move along this edge to both sides of the chipholder. Afterwards, make sure the chip holder is well aligned (edge parallel to the movement)") -> ()  [unwired: 1 in, 1 out]
                  }
                  frame "Set Increment" {
                    n196 = flat-sequence {
                      tunnel: [c_ShowCorner_States."First Move Right"] -> w302
                      frame #0 {
                        # "Set stepsize to move along the \nedge of the chipholder"
                        n197 = global read "g_CipHolderConstants.vi" "Width X"() -> (w305:dbl)
                        n198 = Divide(x=w305, y=2.0) -> (x/y=w303:dbl)
                        n199 = global write "g_CommandParam.vi" "Command"(c_InstructionEnum."Set Stepsize" ("Command")) -> ()
                        n200 = global write "g_CommandParam.vi" "X Stepsize"(w303) -> ()
                      }
                      frame #1 {
                        n201 = Wait (ms)(milliseconds to wait=u32 100) -> ()  [unwired: 1 out]
                      }
                      frame #2 {
                        n202 = call "send_go.vi"() -> ()  [unwired: 12 in]
                      }
                    }
                  }
                  frame "First Move Right" {
                    # "Move from the middle of the top\nedge to the right side and wait until\nmovement is done"
                    n203 = flat-sequence {
                      frame #0 {
                        n204 = global write "g_CommandParam.vi" "Y Steps"(0.0 ("Y Stepsize")) -> ()
                        n205 = global write "g_CommandParam.vi" "X Steps"(1.0 ("X Stepsize")) -> ()
                        n206 = global write "g_CommandParam.vi" "Command"(c_InstructionEnum."Increment" ("Command")) -> ()
                      }
                      frame #1 {
                        n207 = Wait (ms)(milliseconds to wait=u32 100) -> ()  [unwired: 1 out]
                      }
                      frame #2 {
                        n208 = call "send_go.vi"() -> ()  [unwired: 12 in]
                      }
                      frame #3 {
                        n209 = Wait (ms)(milliseconds to wait=u32 500) -> ()  [unwired: 1 out]
                      }
                      frame #4 {
                        n210 = call "PS_Ready.vi"("WaitForReady"=TRUE) -> ()  [unwired: 10 in, 1 out]
                      }
                    }
                  }
                  frame "Move Right" {
                    # "Move from left side to the right side along\nthe top edge and wait until the movement is \ndone"
                    n211 = flat-sequence {
                      frame #0 {
                        n212 = global write "g_CommandParam.vi" "Y Steps"(0.0 ("Y Stepsize")) -> ()
                        n213 = global write "g_CommandParam.vi" "X Steps"(2.0 ("X Stepsize")) -> ()
                        n214 = global write "g_CommandParam.vi" "Command"(c_InstructionEnum."Increment" ("Command")) -> ()
                      }
                      frame #1 {
                        n215 = Wait (ms)(milliseconds to wait=u32 100) -> ()  [unwired: 1 out]
                      }
                      frame #2 {
                        n216 = call "send_go.vi"() -> ()  [unwired: 12 in]
                      }
                      frame #3 {
                        n217 = Wait (ms)(milliseconds to wait=u32 1000) -> ()  [unwired: 1 out]
                      }
                      frame #4 {
                        n218 = call "PS_Ready.vi"("WaitForReady"=TRUE) -> ()  [unwired: 10 in, 1 out]
                      }
                    }
                  }
                  frame "Move Left" {
                    # "Move from right side to the left side along\nthe top edge and wait until the movement is \ndone"
                    n219 = flat-sequence {
                      frame #0 {
                        n220 = global write "g_CommandParam.vi" "Y Steps"(0.0 ("Y Stepsize")) -> ()
                        n221 = global write "g_CommandParam.vi" "X Steps"(-2.0 ("X Stepsize")) -> ()
                        n222 = global write "g_CommandParam.vi" "Command"(c_InstructionEnum."Increment" ("Command")) -> ()
                      }
                      frame #1 {
                        n223 = Wait (ms)(milliseconds to wait=u32 100) -> ()  [unwired: 1 out]
                      }
                      frame #2 {
                        n224 = call "send_go.vi"() -> ()  [unwired: 12 in]
                      }
                      frame #3 {
                        n225 = Wait (ms)(milliseconds to wait=u32 1000) -> ()  [unwired: 1 out]
                      }
                      frame #4 {
                        n226 = call "PS_Ready.vi"("WaitForReady"=TRUE) -> ()  [unwired: 10 in, 1 out]
                      }
                    }
                  }
                  frame "Confirm" {
                    # "Ask user if movement should be repeated.\nIf no quit \"Show Corners\" State Machine"
                    n227 = Two Button Dialog(message="Is the Chipholder well aligned? If no, adjust it and move again.", 1:"No, move again!" ("F button name (\"Cancel\")"), 2:"Yes" ("T button name (\"OK\")")) -> (T button?=w331:bool)
                    n228 = Select(t=c_ShowCorner_States."Confirm", s=w331, f=c_ShowCorner_States."Move Right") -> (s? t:f=w330:T11)
                  }
                }
                n229 = local read "stop"() -> (w296:bool)
                n230 = global read "g_Stop.vi" "STOP"() -> (w295:bool)
                n231 = Compound Arithmetic op=OR(w293, w296, w295) -> (w294:bool)
              }
            }
            frame "Find Reference" {
              n232 = while {
                shift-right: [w353] -> _
                shift-left: c_FindReference_States."Move to Side" -> [w354]
                tunnel: w340 -> [w349]
                tunnel: w341 -> [w348]
                tunnel: [w347] -> w338
                tunnel: [w346] -> w337
                stop <- w352 stop-if-true
                # "Find Reference State Machine"
                n233 = case shown="\"Set Reference\"" w354 {
                  tunnel: [c_FindReference_States."Settings" c_FindReference_States."Find Chipslot" w381 c_FindReference_States."Find Chipslot" c_FindReference_States."Set Reference"] -> w353
                  tunnel: [FALSE _ w380 _ w420] -> w350
                  tunnel: w349 -> [w357 w372 w395 w414 w421]
                  tunnel: w348 -> [w358 w373 w394 w415 w422]
                  tunnel: [w358 w373 w389 w415 w422] -> w347
                  tunnel: [w357 w372 w388 w414 w421] -> w346
                  frame "Move to Side", Default {
                    # "Move from the top left corner of the chipholder to the right side.\n2 mm in Y direction correspond to the distance between the edge \nand the first row of chipslots"
                    n234 = flat-sequence {
                      frame #0 {
                        n235 = Wait (ms)(milliseconds to wait=u32 1) -> ()  [unwired: 1 out]
                      }
                      frame #1 {
                        n236 = global read "g_CipHolderConstants.vi" "Width X"() -> (w361:dbl)
                        n237 = Add(x=w361, y=2.0) -> (x+y=w362:dbl)
                        n238 = global write "g_CommandParam.vi" "Y Stepsize"(0.0 ("Y Stepsize")) -> ()
                        n239 = global write "g_CommandParam.vi" "X Stepsize"(w362) -> ()
                        n240 = global write "g_CommandParam.vi" "Command"(c_InstructionEnum."Set Stepsize" ("Command")) -> ()
                      }
                      frame #2 {
                        n241 = Wait (ms)(milliseconds to wait=u32 300) -> ()  [unwired: 1 out]
                      }
                      frame #3 {
                        n242 = call "send_go.vi"() -> ()  [unwired: 12 in]
                      }
                      frame #4 {
                        n243 = global write "g_CommandParam.vi" "Y Steps"(-1.0 ("Y Stepsize")) -> ()
                        n244 = global write "g_CommandParam.vi" "X Steps"(1.0 ("X Stepsize")) -> ()
                        n245 = global write "g_CommandParam.vi" "Command"(c_InstructionEnum."Increment" ("Command")) -> ()
                      }
                      frame #5 {
                        n246 = call "send_go.vi"() -> ()  [unwired: 12 in]
                      }
                      frame #6 {
                        n247 = Wait (ms)(milliseconds to wait=u32 1000) -> ()  [unwired: 1 out]
                      }
                      frame #7 {
                        n248 = call "PS_Ready.vi"("WaitForReady"=TRUE) -> ()  [unwired: 10 in, 1 out]
                      }
                    }
                  }
                  frame "Settings" {
                    n249 = flat-sequence {
                      frame #0 {
                        # "Set Increment step to move back\ntowards chipslot"
                        n250 = global write "g_CommandParam.vi" "Y Stepsize"(0.1 ("Y Stepsize")) -> ()
                        n251 = global write "g_CommandParam.vi" "X Stepsize"(0.1 ("X Stepsize")) -> ()
                        n252 = global write "g_CommandParam.vi" "Command"(c_InstructionEnum."Set Stepsize" ("Command")) -> ()
                      }
                      frame #1 {
                        n253 = call "send_go.vi"() -> ()  [unwired: 12 in]
                      }
                      frame #2 {
                        # "Set Image Busy for\nImage Processing\nSet Counter for \nDetection Verification\nto zero"
                        n254 = global write "g_GPCounters.vi" "Counter 1"(0.0 ("Counter 1")) -> ()
                        n255 = global write "g_GPCounters.vi" "Counter 2"(0.0 ("Counter 2")) -> ()
                        n256 = local write "ImageBusy"(TRUE ("ImageBusy")) -> ()
                      }
                    }
                  }
                  frame "Find Chipslot" {
                    # "Stops the Loop when more than 40 moves executed"
                    # "Image Analysis to detect the Chipslot"
                    n257 = call "GetInspectionResults.vi"("Select Inspection"=c_VBAI_SelcectInspection."Find Reference", "Image Step Name (default last image used by inspection)"=cluster{"State Name":string, "Step Name":string} {"State Name"="Variable", "Step Name"="IMG_ChipholderCorner"}, "error in (no error)"=w395, "StepName"="Match Pattern Chipholder Corner", "Image Enable"=TRUE, "Refnum in"=w394) -> ("error out"=w388:errorcluster, "Results"=w387:T14, "Image Dst Out"=w390:T1, "Refnum out"=w389:T6)  [unwired: 1 in, 1 out]
                    n258 = Unbundle By Name(w387) -> ("PASS/FAIL Flag"=w385:bool)
                    n259 = local write "Image"(w390) -> ()
                    n260 = case shown="True" w385 {
                      tunnel: [c_FindReference_States."Make Step" w404] -> w381
                      frame False {
                        # "No chipslot detected\n-> move a step"
                        n261 = global read "g_GPCounters.vi" "Counter 2"() -> (w401:dbl)
                        n262 = global write "g_GPCounters.vi" "Counter 1"(0.0 ("Counter 1")) -> ()
                        n263 = Increment(x=w401) -> (x+1=w400:dbl)
                        n264 = global write "g_GPCounters.vi" "Counter 2"(w400) -> ()
                      }
                      frame True {
                        # "If chipslot detected -> verify again without moving"
                        n265 = global read "g_GPCounters.vi" "Counter 1"() -> (w407:dbl)
                        n266 = Greater Or Equal?(x=w407, y=2.0) -> (x >= y?=w405:bool)
                        n267 = case shown="True" w405 {
                          tunnel: [c_FindReference_States."Find Chipslot" c_FindReference_States."Set Reference"] -> w404
                          frame False {
                            n268 = global read "g_GPCounters.vi" "Counter 1"() -> (w409:dbl)
                            n269 = Increment(x=w409) -> (x+1=w410:dbl)
                            n270 = global write "g_GPCounters.vi" "Counter 1"(w410) -> ()
                          }
                          frame True {
                            n271 = global write "g_GPCounters.vi" "Counter 1"(0.0 ("Counter 1")) -> ()
                          }
                        }
                      }
                    }
                    n272 = global read "g_GPCounters.vi" "Counter 2"() -> (w382:dbl)
                    n273 = Greater?(x=w382, y=40.0) -> (0:w384:bool)
                    n274 = case shown="True" w384 {
                      tunnel: [FALSE ("stop") w397] -> w380
                      frame False {
                      }
                      frame True {
                        n275 = stacked-sequence {
                          tunnel: [_ w399] -> w397
                          frame #0 {
                            n276 = One Button Dialog(message="Chipholder not found! Click OK and restart the Testprocedure") -> ()  [unwired: 1 in, 1 out]
                          }
                          frame #1 {
                            w399 = TRUE ("stop")
                            n277 = local write "stop"(w399) -> ()
                          }
                        }
                      }
                    }
                  }
                  frame "Make Step" {
                    # "Make a step"
                    n278 = flat-sequence {
                      frame #0 {
                        n279 = global write "g_CommandParam.vi" "Y Steps"(0.0 ("Y Stepsize")) -> ()
                        n280 = global write "g_CommandParam.vi" "X Steps"(-1.0 ("X Stepsize")) -> ()
                        n281 = global write "g_CommandParam.vi" "Command"(c_InstructionEnum."Increment" ("Command")) -> ()
                      }
                      frame #1 {
                        n282 = call "send_go.vi"() -> ()  [unwired: 12 in]
                      }
                      frame #2 {
                        n283 = Wait (ms)(milliseconds to wait=u32 300) -> ()  [unwired: 1 out]
                      }
                    }
                  }
                  frame "Set Reference" {
                    # "Set the actual position as the Home reference point.\nEnd of the \"Find Reference\" State Machine"
                    n284 = flat-sequence {
                      tunnel: [w431] -> w420
                      frame #0 {
                        n285 = call "GetPosition.vi"() -> ("Y"=w426:dbl, "X"=w427:dbl)  [unwired: 10 in]
                        n286 = Subtract(x=w427, y=4.0) -> (x-y=w429:dbl)
                        n287 = Subtract(x=w426, y=4.0) -> (x-y=w428:dbl)
                        n288 = global write "g_CipHolderConstants.vi" "Home X"(w429) -> ()
                        n289 = global write "g_CipHolderConstants.vi" "Home Y"(w428) -> ()
                      }
                      frame #1 {
                        # "Free Image\nfor normal\nDisplay"
                        n290 = local write "ImageBusy"(FALSE ("ImageBusy")) -> ()
                      }
                      frame #2 {
                        # "Test if Set Reference OK"
                        n291 = global read "g_CipHolderConstants.vi" "Home X"() -> (w432:dbl)
                        n292 = Greater Than 0?(x=w432) -> (x > 0?=w431:bool)
                      }
                    }
                  }
                }
                n293 = Wait (ms)(milliseconds to wait=u32 1) -> ()  [unwired: 1 out]
                n294 = local read "stop"() -> (w345:bool)
                n295 = global read "g_Stop.vi" "STOP"() -> (w351:bool)
                n296 = Compound Arithmetic op=OR(w350, w345, w351) -> (w352:bool)
              }
            }
          }
          n297 = Wait (ms)(milliseconds to wait=u32 1) -> ()  [unwired: 1 out]
          n298 = global read "g_Stop.vi" "STOP"() -> (w220:bool)
          n299 = local read "stop"() -> (w219:bool)
          n300 = Compound Arithmetic op=OR(w211, w219, w220) -> (w214:bool)
        }
      }
      frame "Next Slot" {
        (unwired) FALSE
        n301 = stacked-sequence {
          tunnel: [_ _ w479] -> w433
          frame #0 {
            # "Beginning of the Loop (to go through Array in order to \nfing the next Chipslot"
            n302 = local write "LoopBreak"(FALSE ("LoopBreak")) -> ()
          }
          frame #1 {
            # "-> next slot: Occupied T\n Alignment Processed F"
            # "Alignment Processed\nArray: Chips already\ntried to align"
            # "Occupied Array: Chips\nsupposed to test"
            # "Go through arrays"
            n303 = global read "g_CipHolderConstants.vi" "#Slots X"() -> (w437:dbl)
            n304 = global read "g_CipHolderConstants.vi" "#Slots Y"() -> (w438:dbl)
            n305 = for {
              N: w438 -> [_]
              tunnel: w437 -> [w442]
              i -> [w441]
              stop <- w439 stop-if-true
              # "Y Counter"
              n306 = for {
                N: w442 -> [_]
                tunnel: w441 -> [w445]
                shift-right: [w444] -> w439
                shift-left: FALSE -> [_]
                i -> [w446]
                stop <- w444 stop-if-true
                # "If chipslot occupied but\nnot yet aligned -> next\nslot"
                # "X Counter"
                # "Invert X axis to begin with the tests on the top right corner"
                n307 = global read "g_CipHolderConstants.vi" "#Slots X"() -> (w450:dbl)
                n308 = global read "g_ChipData.vi" "Alignment Processed"() -> (w454:bool[][])
                n309 = global read "g_ChipData.vi" "Occupied"() -> (w455:bool[][])
                n310 = Subtract(x=w450, y=1.0) -> (x-y=w449:dbl)
                n311 = Subtract(x=w449, y=w446) -> (x-y=w447:dbl)
                n312 = Index Array(array=w455, index (row)=w445, index (col)=w447) -> (element=w451:bool)
                n313 = Index Array(array=w454, index (row)=w445, index (col)=w447) -> (element=w452:bool)
                n314 = Not(x=w452) -> (.not. x?=w453:bool)
                n315 = And(x=w451, y=w453) -> (x .and. y?=w443:bool)
                n316 = case shown="False" w443 {
                  tunnel: w445 -> [w461 w470]
                  tunnel: w446 -> [w462 w471]
                  tunnel: [FALSE w468] -> w444
                  frame False {
                    w465 = 1.0 ("y")
                    # "If all the chipslots are tested\nSet ChipsComplete flag"
                    n317 = global read "g_CipHolderConstants.vi" "#Slots X"() -> (w467:dbl)
                    n318 = global read "g_CipHolderConstants.vi" "#Slots Y"() -> (w466:dbl)
                    n319 = Subtract(x=w467, y=w465) -> (x-y=w463:dbl)
                    n320 = Subtract(x=w466, y=w465) -> (x-y=w464:dbl)
                    n321 = Equal?(x=w463, y=w462) -> (x = y?=w460:bool)
                    n322 = Equal?(x=w464, y=w461) -> (x = y?=w459:bool)
                    n323 = And(x=w460, y=w459) -> (x .and. y?=→"ChipsComplete":bool)
                    "LoopBreak" <- FALSE ("LoopBreak")
                  }
                  frame True {
                    # "Set next chipslot"
                    n324 = stacked-sequence {
                      tunnel: w471 -> [w473 _]
                      tunnel: w470 -> [w477 _]
                      tunnel: [_ w478] -> w468
                      frame #0 {
                        n325 = global read "g_CipHolderConstants.vi" "#Slots X"() -> (w476:dbl)
                        n326 = global write "g_ChipData.vi" "Active Y"(w477) -> ()
                        n327 = Subtract(x=w476, y=1.0) -> (x-y=w475:dbl)
                        n328 = Subtract(x=w475, y=w473) -> (x-y=w472:dbl)
                        n329 = global write "g_ChipData.vi" "Active X"(w472) -> ()
                      }
                      frame #1 {
                        w478 = TRUE
                        # "Break the for loop to align \nand test this chip"
                        n330 = local write "LoopBreak"(w478) -> ()
                      }
                    }
                    n331 = local write "ChipsComplete"(FALSE ("ChipsComplete")) -> ()
                  }
                }
              }
            }
          }
          frame #2 {
            # "Test why the for loops finshed"
            n332 = local read "LoopBreak"() -> (w480:bool)
            n333 = case shown="True" w480 {
              tunnel: [w481 c_StateMachine_States."Chip Alignment"] -> w479
              frame False {
                n334 = local read "ChipsComplete"() -> (w482:bool)
                n335 = case shown="True" w482 {
                  tunnel: [c_StateMachine_States."Next Slot" c_StateMachine_States."Report"] -> w481
                  frame False {
                    # "Chips not Complete yet\n-> Go to next slot process"
                  }
                  frame True {
                    # "Chips completed\n-> Go to the final report"
                  }
                }
              }
              frame True {
                # "If there is another Chipslot left (Break out of the \nfor loops)"
                # "Write Header with Chipslot Indication in the Report file\nand go ahead to the Chip Alignment"
                n336 = flat-sequence {
                  frame #0 {
                    w495 = "----------------------------------------------------------------------------------\nChip Position:     "  # Header String
                    n337 = global read "g_ChipData.vi" "Active X"() -> (w496:dbl)
                    n338 = global read "g_ChipData.vi" "Active Y"() -> (w493:dbl)
                    n339 = Number To Decimal String(number=w496) -> (decimal integer string=w489:string)  [unwired: 1 in]
                    n340 = Number To Decimal String(number=w493) -> (decimal integer string=w490:string)  [unwired: 1 in]
                    n341 = global read "g_ChipData.vi" "Active Y"() -> (→"Chip Y":dbl)
                    n342 = global read "g_ChipData.vi" "Active X"() -> (→"Chip X":dbl)
                    n343 = Concatenate Strings(w495, " X: ", w489, " Y: ", w490, "\r\n") -> (w491:string)
                    n344 = global write "g_ReportControl.vi" "Report String"(w491) -> ()
                  }
                  frame #1 {
                    n345 = call "report_write_go.vi"() -> ()  [unwired: 12 in]
                  }
                }
              }
            }
          }
        }
      }
      frame "Chip Alignment" {
        n346 = stacked-sequence {
          tunnel: w505 -> [_ _ _ _ _ _ w543 _ w552 _ _ _]
          tunnel: w504 -> [_ _ _ _ _ _ w542 _ w551 _ _ _]
          tunnel: [_ _ _ _ _ _ w541 _ _ _ _ _] -> w503
          tunnel: [_ _ _ _ _ _ w540 _ _ _ _ _] -> w502
          tunnel: [_ _ _ _ _ _ _ _ _ w583 _ _] -> w501
          tunnel: [_ _ _ _ _ _ _ _ _ w581 _ _] -> w500
          frame #0 {
            n347 = Wait (ms)(milliseconds to wait=u32 100) -> ()  [unwired: 1 out]
          }
          frame #1 {
            # "Enable Loop that reads the shared variables for the measurements on the Image"
            # "Move to the calculated chipslot"
            n348 = global read "g_CipHolderConstants.vi" "Length Chipslot"() -> (w527:dbl)
            n349 = global read "g_ChipData.vi" "Active Y"() -> (w528:dbl)
            n350 = global read "g_CipHolderConstants.vi" "Home Y"() -> (w511:dbl)
            n351 = global read "g_ChipData.vi" "Active X"() -> (w524:dbl)
            n352 = global read "g_CipHolderConstants.vi" "Width Chipslot"() -> (w523:dbl)
            n353 = global read "g_CipHolderConstants.vi" "#Slots X"() -> (w525:dbl)
            n354 = global read "g_CipHolderConstants.vi" "Home X"() -> (w514:dbl)
            n355 = Subtract(x=w525, y=w524) -> (x-y=w518:dbl)
            n356 = Subtract(x=w518, y=1.0) -> (x-y=w517:dbl)
            n357 = Multiply(x=w517, y=w523) -> (x*y=w522:dbl)
            n358 = Multiply(x=w528, y=w527) -> (x*y=w526:dbl)
            n359 = Subtract(x=w514, y=0.0) -> (x-y=w512:dbl)
            n360 = Subtract(x=w511, y=0.0) -> (x-y=w509:dbl)
            n361 = global write "g_VBAIMeasurements.vi" "ReadEnable"(TRUE ("SharedVariableReadEnable")) -> ()
            n362 = Subtract(x=w512, y=w522) -> (x-y=w521:dbl)
            n363 = Subtract(x=w509, y=w526) -> (x-y=w520:dbl)
            n364 = global write "g_CommandParam.vi" "Command"(c_InstructionEnum."Move Absolute" ("Command")) -> ()
            n365 = global write "g_CommandParam.vi" "Y"(w520) -> ()
            n366 = global write "g_CommandParam.vi" "X"(w521) -> ()
          }
          frame #2 {
            # "sends Move command"
            n367 = flat-sequence {
              frame #0 {
                n368 = Wait (ms)(milliseconds to wait=u32 100) -> ()  [unwired: 1 out]
              }
              frame #1 {
                n369 = call "send_go.vi"() -> ()  [unwired: 12 in]
              }
            }
          }
          frame #3 {
            # "Wait during movement"
            n370 = Wait (ms)(milliseconds to wait=u32 1000) -> ()  [unwired: 1 out]
          }
          frame #4 {
            # "Wait until probestation is ready again"
            n371 = call "PS_Ready.vi"("WaitForReady"=TRUE) -> ()  [unwired: 10 in, 1 out]
          }
          frame #5 {
            # "Prepare Image Processing\n- Set Image Busy variable\n- Reset counter"
            n372 = local write "ImageBusy"(TRUE ("ImageBusy")) -> ()
            n373 = global write "g_GPCounters.vi" "Counter 1"(0.0 ("Counter 1")) -> ()
          }
          frame #6 {
            # "Alignment VI"
            # "Update Success Alignment Array in g_ChipData.vi"
            n374 = call "AlignmentProc.vi"("error in (no error)"=w542, "Refnum in"=w543) -> ("error out"=w540:errorcluster, "Image Dst Out"=w534:T1, "Alignment Successful"=w535:bool, "Refnum out"=w541:T6)  [unwired: 6 in]
            "Alignment Successful" <- w535
            n375 = local write "Image"(w534) -> ()
            n376 = global read "g_ChipData.vi" "Success Alignment"() -> (w536:bool[][])
            n377 = global read "g_ChipData.vi" "Active X"() -> (w537:dbl)
            n378 = global read "g_ChipData.vi" "Active Y"() -> (w538:dbl)
            n379 = Replace Array Subset(array=w536, new element=w535, index (row)=w538, index (col)=w537) -> (w539:bool[][])
            n380 = global write "g_ChipData.vi" "Success Alignment"(w539) -> ()
          }
          frame #7 {
            # "Stop the Loop that reads the shared variables"
            # "Free Image for normal Display"
            # "Update Alignement Processed Array in g_ChipData.vi that indicates that the Alignment was processed, even when not successful"
            n381 = global read "g_ChipData.vi" "Alignment Processed"() -> (w545:bool[][])
            n382 = local write "ImageBusy"(FALSE ("ImageBusy")) -> ()
            n383 = global read "g_ChipData.vi" "Active X"() -> (w546:dbl)
            n384 = global read "g_ChipData.vi" "Active Y"() -> (w547:dbl)
            n385 = global write "g_VBAIMeasurements.vi" "ReadEnable"(FALSE ("SharedVariableReadEnable")) -> ()
            n386 = Replace Array Subset(array=w545, new element=TRUE ("new element/subarray"), index (row)=w547, index (col)=w546) -> (w549:bool[][])
            n387 = global write "g_ChipData.vi" "Alignment Processed"(w549) -> ()
          }
          frame #8 {
            # "If the automatic Alignment Process\nwas succssfull, let the user make \ncorrections with Keyboard\nand wait for confirmation"
            n388 = local read "Alignment Successful"() -> (w553:bool)
            n389 = case shown="True" w553 {
              tunnel: w552 -> [_ w555]
              tunnel: w551 -> [_ w554]
              frame False {
              }
              frame True {
                n390 = flat-sequence {
                  tunnel: w555 -> [w569]
                  tunnel: w554 -> [w568]
                  frame #0 {
                    n391 = property on="BrightnessAdjustment" class="Bool (strict)"("Visible"=TRUE, "DisabledEnum"=T3."Enabled" ("Disabled")) -> ()  [unwired: 2 in, 2 out]
                    n392 = property on="ConfirmAlignment" class="Bool (strict)"("Visible"=TRUE, "DisabledEnum"=T3."Enabled" ("Disabled"), "Key Focus"=TRUE) -> ()  [unwired: 2 in, 2 out]
                    n393 = property on="CancelAlignment" class="Bool (strict)"("Visible"=TRUE, "DisabledEnum"=T3."Enabled" ("Disabled")) -> ()  [unwired: 2 in, 2 out]
                    n394 = property on="RedoAlignment" class="Bool (strict)"("Visible"=TRUE, "DisabledEnum"=T3."Enabled" ("Disabled")) -> ()  [unwired: 2 in, 2 out]
                    n395 = global write "g_CommandParam.vi" "X Stepsize"(0.005 ("X Stepsize")) -> ()
                    n396 = global write "g_CommandParam.vi" "Y Stepsize"(0.005 ("Y Stepsize")) -> ()
                    n397 = global write "g_CommandParam.vi" "Command"(c_InstructionEnum."Set Stepsize" ("Command")) -> ()
                  }
                  frame #1 {
                    n398 = call "send_go.vi"() -> ()  [unwired: 12 in]
                  }
                  frame #2 {
                    n399 = while {
                      tunnel: w569 -> [w576]
                      tunnel: w568 -> [w575]
                      stop <- w573 stop-if-true
                      n400 = local read "BrightnessAdjustment"() -> (w574:bool)
                      n401 = local read "ConfirmAlignment"() -> (w571:bool)
                      n402 = local read "CancelAlignment"() -> (w572:bool)
                      n403 = local read "RedoAlignment"() -> (w570:bool)
                      n404 = case shown="True" w574 {
                        tunnel: w576 -> [_ w580]
                        tunnel: w575 -> [_ w579]
                        frame False {
                        }
                        frame True {
                          n405 = local write "BrightnessAdjustment"(FALSE ("BrightnessAdjustment")) -> ()
                          n406 = call "BrightnessSettings.vi"("error in (no error)"=w579, "Refnum in"=w580) -> ()  [unwired: 8 in, 2 out]
                        }
                      }
                      n407 = Compound Arithmetic op=OR(w572, w571, w570) -> (w573:bool)
                      n408 = Wait (ms)(milliseconds to wait=u32 100) -> ()  [unwired: 1 out]
                    }
                  }
                }
              }
            }
          }
          frame #9 {
            # "Write results of the \nAlignement in the arrays\nand in the report"
            n409 = local read "Alignment Successful"() -> (w582:bool)
            n410 = case shown="True" w582 {
              tunnel: [w584 w587] -> w583
              tunnel: [w584 w585] -> w581
              frame False {
                w584 = FALSE
              }
              frame True {
                n411 = local read "RedoAlignment"() -> (w586:bool)
                n412 = local read "ConfirmAlignment"() -> (w588:bool)
                n413 = local read "CancelAlignment"() -> (w589:bool)
                n414 = case shown="True" w586 {
                  tunnel: [FALSE w591] -> w585
                  frame False {
                  }
                  frame True {
                    n415 = flat-sequence {
                      tunnel: [TRUE] -> w591
                      frame #0 {
                        n416 = global write "g_ReportControl.vi" "Report String"(T13 "Chip Realignment Requested" ("Combo Box")) -> ()
                      }
                      frame #1 {
                        n417 = Wait (ms)(milliseconds to wait=u32 2) -> ()  [unwired: 1 out]
                      }
                      frame #2 {
                        n418 = call "report_write_go.vi"() -> ()  [unwired: 12 in]
                      }
                      frame #3 {
                      }
                    }
                  }
                }
                n419 = case shown="True" w589 {
                  frame False {
                  }
                  frame True {
                    n420 = flat-sequence {
                      frame #0 {
                        n421 = global read "g_ChipData.vi" "Success Alignment"() -> (w606:bool[][])
                        n422 = global read "g_ChipData.vi" "Active X"() -> (w607:dbl)
                        n423 = global read "g_ChipData.vi" "Active Y"() -> (w608:dbl)
                        n424 = Replace Array Subset(array=w606, new element=FALSE ("new element/subarray"), index (row)=w608, index (col)=w607) -> (w609:bool[][])
                        n425 = global write "g_ChipData.vi" "Success Alignment"(w609) -> ()
                      }
                      frame #1 {
                        n426 = global write "g_ReportControl.vi" "Report String"(T13 "Chip Alignment Canceled" ("Combo Box")) -> ()
                      }
                      frame #2 {
                        n427 = Wait (ms)(milliseconds to wait=u32 2) -> ()  [unwired: 1 out]
                      }
                      frame #3 {
                        n428 = call "report_write_go.vi"() -> ()  [unwired: 12 in]
                      }
                    }
                  }
                }
                n429 = case shown="True" w588 {
                  tunnel: [FALSE w596] -> w587
                  frame False {
                  }
                  frame True {
                    n430 = flat-sequence {
                      tunnel: [TRUE] -> w596
                      frame #0 {
                        n431 = global read "g_ChipData.vi" "Success Alignment"() -> (w598:bool[][])
                        n432 = global read "g_ChipData.vi" "Active X"() -> (w599:dbl)
                        n433 = global read "g_ChipData.vi" "Active Y"() -> (w600:dbl)
                        n434 = Replace Array Subset(array=w598, new element=TRUE ("new element/subarray"), index (row)=w600, index (col)=w599) -> (w601:bool[][])
                        n435 = global write "g_ChipData.vi" "Success Alignment"(w601) -> ()
                      }
                      frame #1 {
                        n436 = global write "g_ReportControl.vi" "Report String"(T13 "Chip Alignment Successful" ("Combo Box")) -> ()
                      }
                      frame #2 {
                        n437 = Wait (ms)(milliseconds to wait=u32 2) -> ()  [unwired: 1 out]
                      }
                      frame #3 {
                        n438 = call "report_write_go.vi"() -> ()  [unwired: 12 in]
                      }
                      frame #4 {
                      }
                    }
                  }
                }
              }
            }
          }
          frame #10 {
            n439 = local read "ConfirmAlignment"() -> (w615:bool)
            n440 = local read "CancelAlignment"() -> (w614:bool)
            n441 = Not(x=w614) -> (.not. x?=w613:bool)
            n442 = Compound Arithmetic op=AND("Move Plate", w615, w613) -> (w616:bool)
            n443 = case shown="True" w616 {
              frame False {
              }
              frame True {
                n444 = flat-sequence {
                  frame #0 {
                    n445 = global write "g_CommandParam.vi" "Plate Position"(c_PlatePosEnum."Contact" ("Plate Position")) -> ()
                    n446 = global write "g_CommandParam.vi" "Command"(c_InstructionEnum."Move Plate" ("Command")) -> ()
                  }
                  frame #1 {
                    n447 = call "send_go.vi"() -> ()  [unwired: 12 in]
                  }
                  frame #2 {
                    n448 = Wait (ms)(milliseconds to wait=u32 2000) -> ()  [unwired: 1 out]
                  }
                  frame #3 {
                    n449 = global write "g_CommandParam.vi" "Plate Position"(c_PlatePosEnum."Seperate" ("Plate Position")) -> ()
                    n450 = global write "g_CommandParam.vi" "Command"(c_InstructionEnum."Move Plate" ("Command")) -> ()
                  }
                  frame #4 {
                    n451 = call "send_go.vi"() -> ()  [unwired: 12 in]
                  }
                  frame #5 {
                    n452 = Wait (ms)(milliseconds to wait=u32 2000) -> ()  [unwired: 1 out]
                  }
                  frame #6 {
                    n453 = global write "g_CommandParam.vi" "Plate Position"(c_PlatePosEnum."Contact" ("Plate Position")) -> ()
                    n454 = global write "g_CommandParam.vi" "Command"(c_InstructionEnum."Move Plate" ("Command")) -> ()
                  }
                  frame #7 {
                    n455 = call "send_go.vi"() -> ()  [unwired: 12 in]
                  }
                  frame #8 {
                    n456 = Wait (ms)(milliseconds to wait=u32 2000) -> ()  [unwired: 1 out]
                  }
                }
              }
            }
          }
          frame #11 {
            # "Hide Confirm Buttons again and reset flags"
            n457 = local write "ConfirmAlignment"(FALSE ("ConfirmAlignment")) -> ()
            n458 = local write "CancelAlignment"(FALSE ("ConfirmAlignment")) -> ()
            n459 = local write "RedoAlignment"(FALSE) -> ()
            n460 = property on="ConfirmAlignment" class="Bool (strict)"("Visible"=FALSE, "DisabledEnum"=T3."Disabled" ("Disabled"), "Key Focus"=FALSE) -> ()  [unwired: 2 in, 2 out]
            n461 = property on="CancelAlignment" class="Bool (strict)"("Visible"=FALSE, "DisabledEnum"=T3."Disabled" ("Disabled")) -> ()  [unwired: 2 in, 2 out]
            n462 = property on="RedoAlignment" class="Bool (strict)"("Visible"=FALSE, "DisabledEnum"=T3."Disabled" ("Disabled")) -> ()  [unwired: 2 in, 2 out]
            n463 = local write "BrightnessAdjustment"(FALSE ("CancelAlignment")) -> ()
            n464 = property on="BrightnessAdjustment" class="Bool (strict)"("Visible"=FALSE, "DisabledEnum"=T3."Disabled" ("Disabled")) -> ()  [unwired: 2 in, 2 out]
          }
        }
        n465 = Select(t=c_StateMachine_States."Test", s=w501, f=c_StateMachine_States."Next Slot") -> (s? t:f=w498:T2)
        n466 = Select(t=c_StateMachine_States."Chip Alignment", s=w500, f=w498) -> (s? t:f=w499:T2)
      }
      frame "Test" {
        n467 = flat-sequence {
          tunnel: [c_StateMachine_States."Next Slot"] -> w639
          frame #0 {
            # "HCC Test"
            n468 = call "HCCTest.vi"() -> ()  [unwired: 12 in]
          }
          frame #1 {
            n469 = while {
              stop <- w642 stop-if-true
              n470 = One Button Dialog(message="Done testing. Proceed to next?", button name ("OK")="Yep") -> (true=w642:bool)
            }
          }
          frame #2 {
            n471 = global write "g_CommandParam.vi" "Plate Position"(c_PlatePosEnum."Seperate" ("Plate Position")) -> ()
            n472 = global write "g_CommandParam.vi" "Command"(c_InstructionEnum."Move Plate" ("Command")) -> ()
          }
          frame #3 {
            n473 = call "send_go.vi"() -> ()  [unwired: 12 in]
          }
          frame #4 {
          }
        }
      }
      frame "Report" {
        (unwired) FALSE
        n474 = global read "g_ReportControl.vi" "Report Enable"() -> (w649:bool)
        n475 = case shown="True" w649 {
          tunnel: [w652 w653] -> _
          frame False {
            # "If report was disabled, just show Testresult display"
            n476 = call "ShowTestresult.vi"() -> ("Terminated"=w652:bool)  [unwired: 11 in]
          }
          frame True {
            # "If report was enabled, show report file and testresult diplay window"
            n477 = flat-sequence {
              tunnel: [w655] -> w654
              tunnel: [w660] -> w653
              tunnel: w654 -> [w660]
              frame #0 {
                n478 = call "ShowTestresult.vi"() -> ("Terminated"=w655:bool)  [unwired: 11 in]
              }
              frame #1 {
                n479 = global read "g_ReportControl.vi" "selected path"() -> (w658:path)
                n480 = Path To String(path=w658) -> (string=w656:string)
                n481 = Concatenate Strings("notepad " ("string"), w656) -> (w659:string)
                n482 = call <vilib>:"System Exec.vi"("command line"=w659) -> ()  [unwired: 7 in, 4 out]
              }
            }
          }
        }
      }
      frame "End" {
        (unwired) FALSE
        n483 = local write "stop"(TRUE ("stop")) -> ()
      }
    }
    n484 = Wait (ms)(milliseconds to wait=u32 1) -> ()  [unwired: 1 out]
    n485 = global read "g_Stop.vi" "STOP"() -> (w57:bool)
    n486 = local read "stop"() -> (w51:bool)
    n487 = local read "stop"() -> (w50:bool)
    n488 = global write "g_Stop.vi" "TestProcSTOP"(w50) -> ()
    n489 = Compound Arithmetic op=OR(w57, w51) -> (w56:bool)
    "Actual State" <- w48
  }
  n490 = while {
    tunnel: w16 -> [w674]
    stop <- w665 stop-if-true
    # "Parallel Loop for Image Display"
    n491 = global read "g_Stop.vi" "STOP"() -> (w671:bool)
    n492 = local read "stop"() -> (w667:bool)
    n493 = global read "g_Stop.vi" "STOP"() -> (w675:bool)
    n494 = local read "stop"() -> (w670:bool)
    n495 = Compound Arithmetic op=OR("ImageBusy", w667, w671) -> (w672:bool)
    n496 = case shown="False" w672 {
      tunnel: w674 -> [w681 _]
      frame False {
        n497 = call "GetInspectionResults.vi"("Select Inspection"=c_VBAI_SelcectInspection."Image Acquisition", "Image Step Name (default last image used by inspection)"=cluster{"State Name":string, "Step Name":string} {"State Name"="Variable", "Step Name"="IMG_CameraAcquisition"}, "Image Enable"=TRUE, "Refnum in"=w681) -> ("Image Dst Out"=w683:T1)  [unwired: 3 in, 4 out]
        n498 = local write "Image"(w683) -> ()
      }
      frame True {
        # "Image in use for processing"
      }
    }
    n499 = local write "stop"("stop") -> ()
    n500 = Compound Arithmetic op=OR(w675, w670) -> (w668:bool)
    n501 = case shown="False" w668 {
      selector: w668 -> [w676 w677]
      tunnel: [w676 w677] -> w665
      frame False {
      }
      frame True {
        n502 = global write "g_ReportControl.vi" "Report Enable"(FALSE ("Report Enable")) -> ()
      }
    }
    n503 = Wait (ms)(milliseconds to wait=u32 1) -> ()  [unwired: 1 out]
  }
  n504 = while {
    stop <- w686 stop-if-true
    # "Wait to start report loop"
    n505 = global read "g_ReportControl.vi" "New Report"() -> (w684:bool)
    n506 = case shown="False" w684 {
      frame False {
        n507 = Wait (ms)(milliseconds to wait=u32 10) -> ()  [unwired: 1 out]
      }
      frame True {
        n508 = call "Report.vi"() -> ()  [unwired: 12 in]
      }
    }
    n509 = global read "g_Stop.vi" "STOP"() -> (w687:bool)
    n510 = local read "stop"() -> (w685:bool)
    n511 = Compound Arithmetic op=OR(w687, w685) -> (w686:bool)
  }
  n512 = flat-sequence {
    tunnel: w18 -> [w690]
    tunnel: w19 -> [w691]
    tunnel: [w691] -> w15
    tunnel: [w690] -> w14
    tunnel: w15 -> [w693]
    tunnel: w14 -> [w692]
    frame #0 {
      n513 = Wait (ms)(milliseconds to wait=u32 200) -> ()  [unwired: 1 out]
    }
    frame #1 {
      # "Close Vision Builder"
      n514 = call <vilib>:"VBAI Interface - Stop Inspection.vi"("error in"=w692, "Session In"=w693) -> ("error out"=w694:errorcluster, "Session Out"=w695:T6)  [unwired: 8 in]
      n515 = call <vilib>:"VBAI Interface - Close Connection.vi"("error in"=w694, "Session In"=w695) -> ("error out"=w696:errorcluster)  [unwired: 9 in]
      n516 = call "IMAQ Dispose"("All Images? (No)"=TRUE, "error in (no error)"=w696) -> ()  [unwired: 4 in, 1 out]
    }
  }
